vi "read_cmd_response.vi"(8 "error in (no error)":errorcluster, 10 "command response":string) -> (0 "error out":errorcluster, 1 "response":string, 2 "acknowledged?":bool)   [LabVIEW 2018, in "Inficon IC6.lvlib"]
doc: "Read the elements of a command response packet."
uses:
  <instrlib>/Inficon IC6/Inficon IC6.lvlib
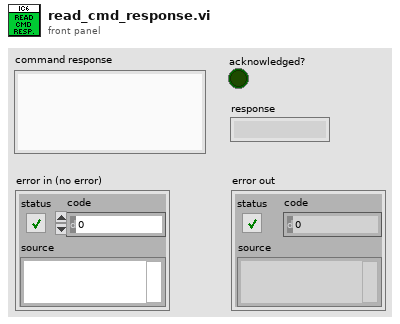
[diagram p1: front panel]
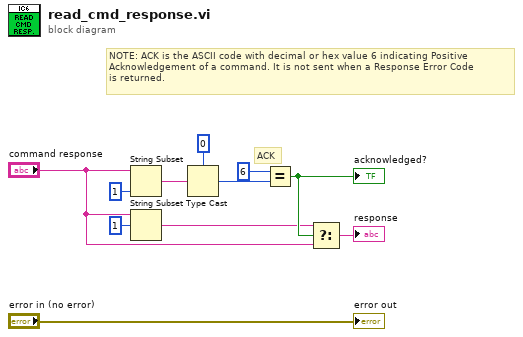
[diagram p0: block diagram]
diagram:
  # "NOTE: ACK is the ASCII code with decimal or hex value 6 indicating Positive\nAcknowledgement of a command. It is not sent when a Response Error Code\nis returned."
  # "ACK"
  n1 = String Subset(string="command response", length (rest)=1 ("length (rest)")) -> (substring=w8:string)  [unwired: 1 in]
  n2 = String Subset(string="command response", offset (0)=1 ("length (rest)")) -> (substring=w3:string)  [unwired: 1 in]
  n3 = Type Cast(type=u8 0 ("x"), x=w8) -> (*(type *) &x=w10:u8)
  n4 = Equal?(x=u8 6, y=w10) -> (x = y?=w4:bool)
  "acknowledged?" <- w4
  n5 = Select(t=w3, s=w4, f="command response") -> (s? t:f=→"response":string)
  "error out" <- "error in (no error)"
